vi "StringifiedData.vi"(8 "error in (no error)":errorcluster, 11 "I32Msg in":refnum<class "I32Msg.lvclass">) -> (0 "error out":errorcluster, 2 "Stringified Data":string, 3 "I32Msg out":refnum<class "I32Msg.lvclass">)   [LabVIEW 2013, in "LapDog.Messaging.v3.NativeTypes.lvlib" / "I32Msg.lvclass"]
doc: "This VI is used for the message probe. Child classes may override it and provide the message data in string format or a short string describing the data the message contains. This string will be displayed in the probe window."
uses:
  I32Msg.lvclass
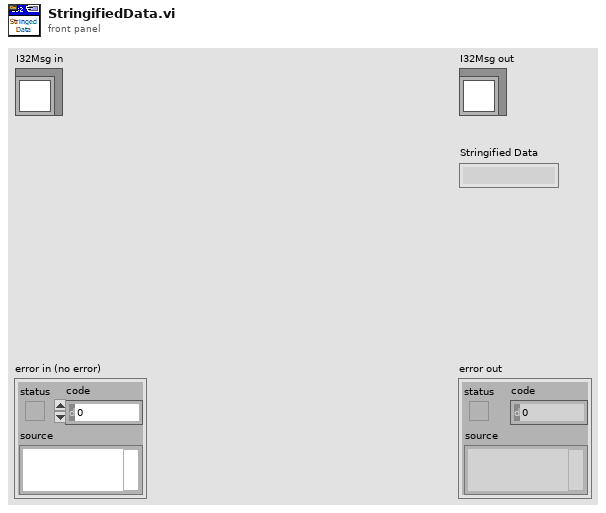
[diagram p1: front panel]
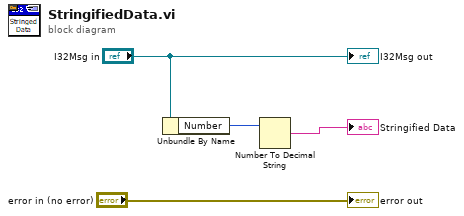
[diagram p0: block diagram]
diagram:
  n1 = Unbundle By Name("I32Msg in") -> ("Number"=w1:i32)
  n2 = Number To Decimal String(number=w1) -> (decimal integer string=→"Stringified Data":string)  [unwired: 1 in]
  "error out" <- "error in (no error)"
  "I32Msg out" <- "I32Msg in"
